vi "run.vi"(8 "error in (no error)":errorcluster, 11 "ScanHeadAK130114ResonanceFlexRIO in":refnum<class "ScanHeadAK130114ResonanceFlexRIO.lvclass">) -> (0 "error out":errorcluster, 3 "ScanHeadAK130114ResonanceFlexRIO out":refnum<class "ScanHeadAK130114ResonanceFlexRIO.lvclass">)   [LabVIEW 2010, in "ScanHeadAK130114ResonanceFlexRIO.lvclass"]
uses:
  ScanHeadAK130114ResonanceFlexRIO.lvclass
  GenericScanHead/GenericScanHead/GenericScanHead.lvclass
  common/classes/ErrorController/ErrorController/ErrorController.lvclass
  Trajectory/GenericTrajectory/GenericTrajectory/GenericTrajectory.lvclass
  internal_trigger_enum.ctl
  main/labview_source/controls/undock_button.ctl
panel:
  in  "button:undock":T1
  in  "Tab Control":enum32{"user", "debug", "about"}(tab)
  in  "number of pulses":u16(ring) items=["0", "1", "2"]
  in  "duration of pulse 2":dbl[unit]
  in  "offset to pulse 2":dbl[unit]
  in  "duration of pulse 1":dbl[unit]
  in  "offset to pulse 1":dbl[unit]
  in  "offset fly back":dbl(slide)=55.301 min=0.001 max=100.0 step=0.1 scale=0.0..100.0
  in  "offset fly forward":dbl(slide)=26.401 min=0.001 max=100.0 step=0.1 scale=0.0..100.0
  in  "scan segment":dbl(slide)=50.001000000000005 min=0.001 max=100.0 step=0.1 scale=0.0..100.0
  in  "modifyButton":bool
  in  "zoom":dbl(slide)=1.5 min=1.0 max=20.0 step=0.1 scale=1.0..20.0
  in  "laser intensity":dbl(slide)=14.5 caption="intensity" min=0.001 max=100.0 step=0.1 scale=0.0..100.0
  in  "stop":bool
  out "event loop error":errorcluster
  out "state machine counter":i32
  out "last trigger":T2
  # "translation"
  # "fov and laser power"
  # "resonance cycle fractions"
  # "ScanHeadAK130114ResonanceFlexRIO"
  # "Author: Andreas Keller, ETH Zurich, Switzerland"
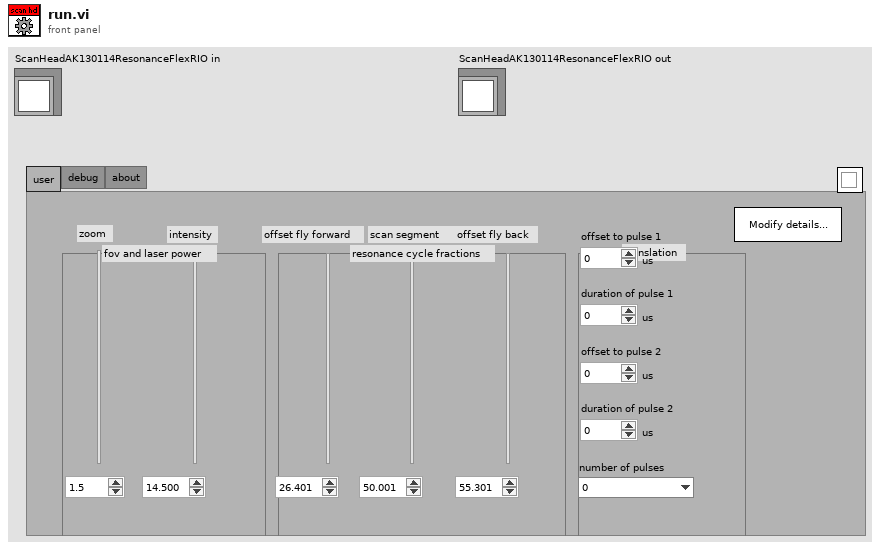
[diagram p1: front panel]
types:
  T1 = typedef "undock_button.ctl" = bool
  T2 = typedef "ScanHeadAK130114ResonanceFlexRIO.lvclass/internal_trigger_enum.ctl" = enum16{"NULL", "initialise", "terminate", "start scanning", "stop scanning", "update", "fetch trajectory"}
  T3 = typedef "top-level_component_type_enum.ctl" = enum16{"undefined", "ImagingMode", "ScanHead", "DAQ", "ImageAssembler", "Display", "DataCollection", "Analyser", "Stimulator", "ExperimentController", "Instrument", "Stage"}
  T4 = typedef "main_trigger_enum.ctl" = enum16{"NULL", "initialise", "terminate", "start", "stop", "change objective", "change experimentController", "change imagingMode", "save notebook", "started saving", "finished saving", "expCtr ready", "expCtr missing", "imgMd ready", "imgMd missing", "scanHd ready", "scanHd missing", "DAQ ready", "DAQ missing", "imgAsm ready", "imgAsm missing", "dataColl ready", "dataColl missing", "display ready", "display missing", "analysr ready", "analysr missing", "instrmnt ready", "instrmnt missing", "stimltr ready", "stimltr missing", "stage ready", "stage missing"}
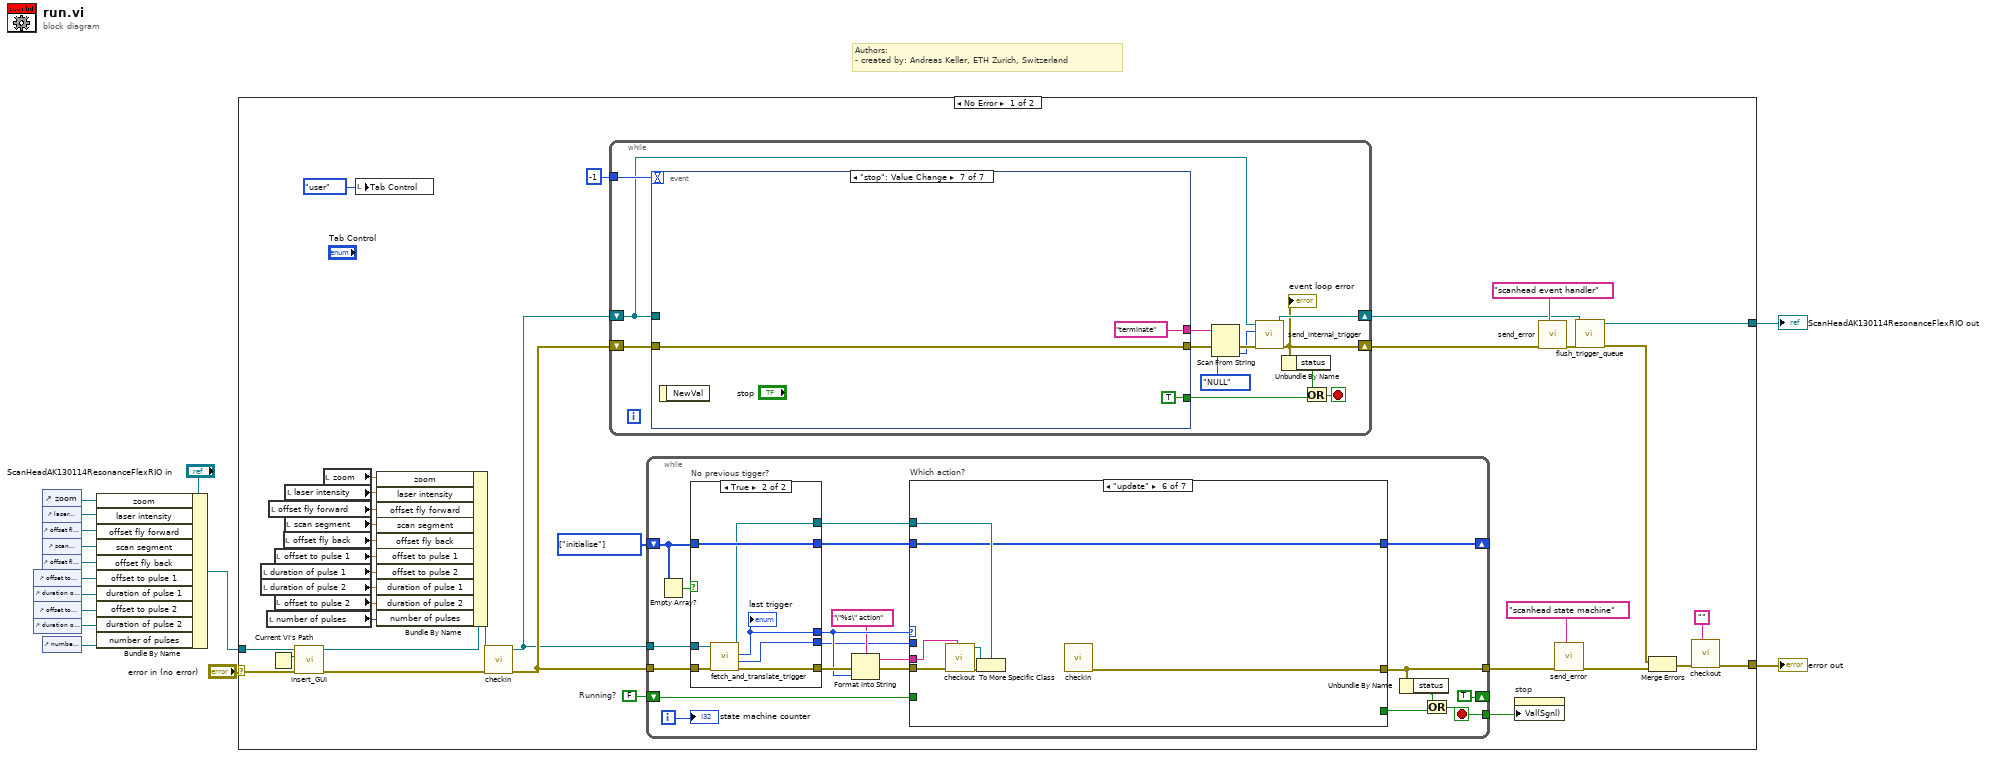
[diagram p0: block diagram]
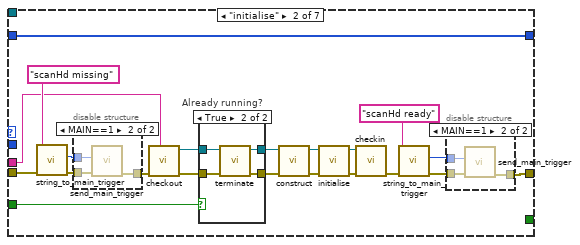
[diagram p3: hidden frame]
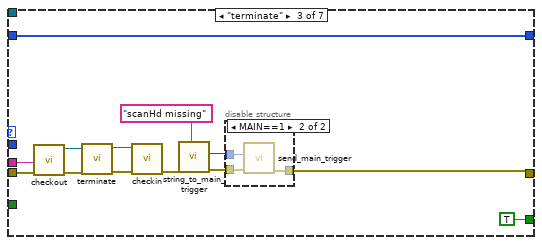
[diagram p7: hidden frame]
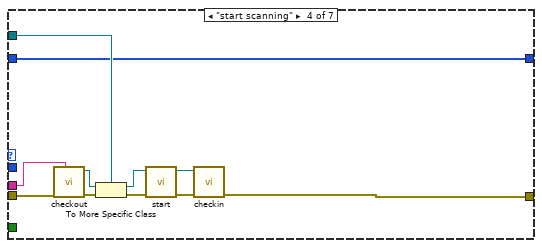
[diagram p9: hidden frame]
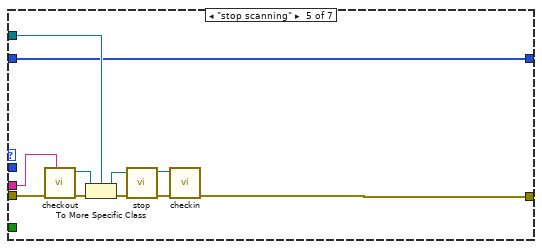
[diagram p10: hidden frame]
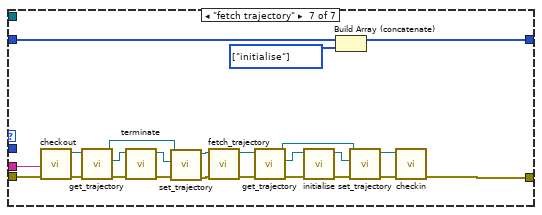
[diagram p11: hidden frame]
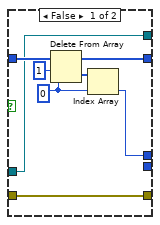
[diagram p12: hidden frame]
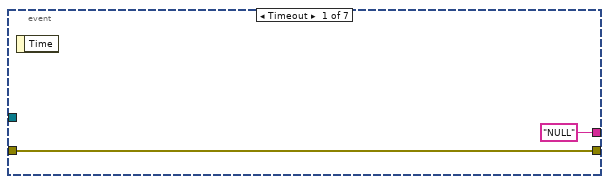
[diagram p13: hidden frame]
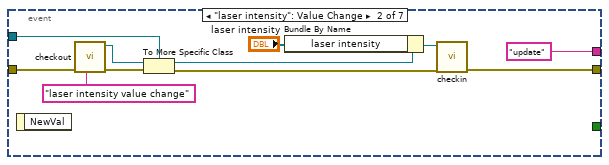
[diagram p14: hidden frame]
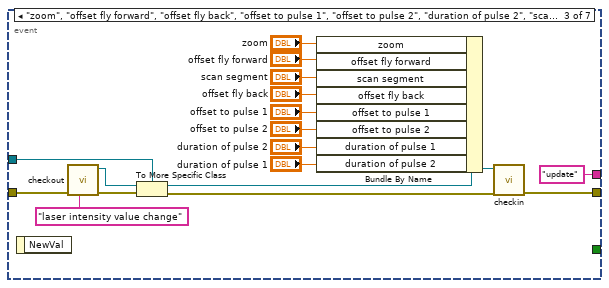
[diagram p15: hidden frame]
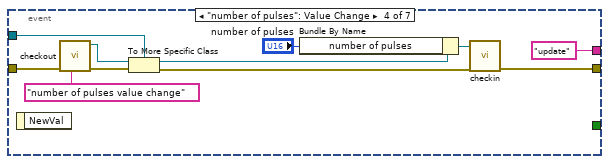
[diagram p16: hidden frame]
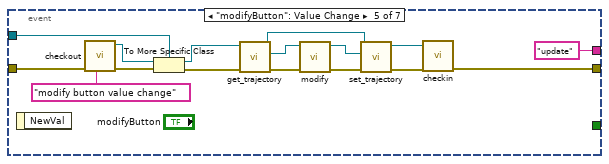
[diagram p17: hidden frame]
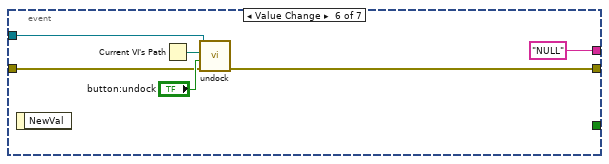
[diagram p18: hidden frame]
diagram:
  # "Authors: \n- created by: Andreas Keller, ETH Zurich, Switzerland"
  n1 = control-ref of="offset to pulse 1"() -> (w6:refnum<vi>)
  n2 = control-ref of="duration of pulse 1"() -> (w5:refnum<vi>)
  n3 = control-ref of="offset to pulse 2"() -> (w4:refnum<vi>)
  n4 = control-ref of="duration of pulse 2"() -> (w3:refnum<vi>)
  n5 = control-ref of="zoom"() -> (w11:refnum<vi>)
  n6 = control-ref of="laser intensity"() -> (w10:refnum<vi>)
  n7 = control-ref of="offset fly forward"() -> (w9:refnum<vi>)
  n8 = control-ref of="scan segment"() -> (w8:refnum<vi>)
  n9 = control-ref of="offset fly back"() -> (w7:refnum<vi>)
  n10 = control-ref of="number of pulses"() -> (w2:refnum<vi>)
  n11 = Bundle By Name(cluster="ScanHeadAK130114ResonanceFlexRIO in", "zoom"=w11, "laser intensity"=w10, "offset fly forward"=w9, "scan segment"=w8, "offset fly back"=w7, "offset to pulse 1"=w6, "duration of pulse 1"=w5, "offset to pulse 2"=w4, "duration of pulse 2"=w3, "number of pulses"=w2) -> (w1:refnum<class "ScanHeadAK130114ResonanceFlexRIO.lvclass">)
  n12 = case shown="No Error" "error in (no error)" {
    selector: "error in (no error)" -> [w48 w273]
    tunnel: w1 -> [w49 w274]
    tunnel: [w27 w274] -> w14
    tunnel: [w24 w273] -> w13
    frame No Error {
      w16 = T2[] [enum."initialise"] items=["NULL", "initialise", "terminate", "start scanning", "stop scanning", "update", "fetch trajectory"]
      w19 = FALSE  # Running?
      n13 = local read "duration of pulse 1"() -> (w40:dbl[unit])
      n14 = local read "duration of pulse 2"() -> (w39:dbl[unit])
      n15 = local read "number of pulses"() -> (w37:u16)
      n16 = local read "offset fly forward"() -> (w44:dbl)
      n17 = Current VI's Path() -> (path=w50:path)
      n18 = local read "offset to pulse 1"() -> (w41:dbl[unit])
      n19 = local read "offset to pulse 2"() -> (w38:dbl[unit])
      n20 = local read "offset fly back"() -> (w42:dbl)
      n21 = local read "scan segment"() -> (w43:dbl)
      n22 = local read "laser intensity"() -> (w45:dbl)
      n23 = call-dynamic "insert_GUI.vi"("error in (no error)"=w48, "VI path"=w50, "GenericComponent in"=w49) -> ("error out"=w36:errorcluster, "GenericComponent out"=w47:refnum<class "ScanHeadAK130114ResonanceFlexRIO.lvclass">)  [unwired: 7 in]
      n24 = local read "zoom"() -> (w46:dbl)
      n25 = local write "Tab Control"(enum32{"user", "debug", "about"}."user" ("Tab Control")) -> ()
      n26 = Bundle By Name(cluster=w47, "zoom"=w46, "laser intensity"=w45, "offset fly forward"=w44, "scan segment"=w43, "offset fly back"=w42, "offset to pulse 1"=w41, "offset to pulse 2"=w40, "duration of pulse 1"=w39, "duration of pulse 2"=w38, "number of pulses"=w37) -> (w35:refnum<class "ScanHeadAK130114ResonanceFlexRIO.lvclass">)
      n27 = call-dynamic "checkin.vi"("error in (no error)"=w36, "GenericScanHead in"=w35) -> ("error out"=w33:errorcluster, "GenericScanHead out"=w32:refnum<class "ScanHeadAK130114ResonanceFlexRIO.lvclass">)  [unwired: 8 in]
      n28 = while {
        tunnel: -1 -> [w205]
        shift-right: [w196] -> w31
        shift-left: w33 -> [w204]
        shift-right: [w198] -> w28
        shift-left: w32 -> [w197]
        stop <- w199 stop-if-true
        n29 = event shown="[6] \"stop\": Value Change" {
          selector: _ -> [_ _ _ _ _ _ _]
          dyn-events: _ -> [_ _ _ _ _ _ _]
          timeout: w205 -> [_ _ _ _ _ _ _]
          tunnel: w204 -> [w206 w211 w232 w238 w261 w267 w272]
          tunnel: [w206 w210 w231 w240 w260 w266 w272] -> w202
          tunnel: ["NULL" "update" "update" "update" "update" "NULL" "terminate"] -> w203
          tunnel: w197 -> [_ w212 w233 w245 w259 w269 _]
          tunnel: [_ _ _ _ _ _ TRUE] -> w194
          event Timeout {
            n30 = event-data() -> ()  [unwired: 1 in, 1 out]
          }
          event "laser intensity": Value Change {
            n31 = event-data() -> ()  [unwired: 1 in, 1 out]
            n32 = call "checkout.vi"("locked by?"="laser intensity value change", "error in (no error)"=w211) -> ("error out"=w216:errorcluster, "GenericScanHead out"=w218:refnum<class "GenericScanHead.lvclass">)  [unwired: 8 in]
            n33 = To More Specific Class(target class=w212, reference=w218, error in=w216) -> (specific class reference=w214:refnum<class "ScanHeadAK130114ResonanceFlexRIO.lvclass">, error out=w215:errorcluster)
            n34 = Bundle By Name(cluster=w214, "laser intensity"="laser intensity") -> (w213:refnum<class "ScanHeadAK130114ResonanceFlexRIO.lvclass">)
            n35 = call-dynamic "checkin.vi"("error in (no error)"=w215, "GenericScanHead in"=w213) -> ("error out"=w210:errorcluster)  [unwired: 8 in, 1 out]
          }
          event "zoom", "offset fly forward", "offset fly back", "offset to pulse 1", "offset to pulse 2", "duration of pulse 2", "scan segment", "duration of pulse 1": Value Change {
            n36 = event-data() -> ()  [unwired: 1 in, 1 out]
            n37 = call "checkout.vi"("locked by?"="laser intensity value change", "error in (no error)"=w232) -> ("error out"=w235:errorcluster, "GenericScanHead out"=w236:refnum<class "GenericScanHead.lvclass">)  [unwired: 8 in]
            n38 = To More Specific Class(target class=w233, reference=w236, error in=w235) -> (specific class reference=w229:refnum<class "ScanHeadAK130114ResonanceFlexRIO.lvclass">, error out=w234:errorcluster)
            n39 = Bundle By Name(cluster=w229, "zoom"="zoom", "offset fly forward"="offset fly forward", "scan segment"="scan segment", "offset fly back"="offset fly back", "offset to pulse 1"="offset to pulse 1", "offset to pulse 2"="offset to pulse 2", "duration of pulse 1"="duration of pulse 2", "duration of pulse 2"="duration of pulse 1") -> (w228:refnum<class "ScanHeadAK130114ResonanceFlexRIO.lvclass">)
            n40 = call-dynamic "checkin.vi"("error in (no error)"=w234, "GenericScanHead in"=w228) -> ("error out"=w231:errorcluster)  [unwired: 8 in, 1 out]
          }
          event "number of pulses": Value Change {
            n41 = event-data() -> ()  [unwired: 1 in, 1 out]
            n42 = call "checkout.vi"("locked by?"="number of pulses value change", "error in (no error)"=w238) -> ("error out"=w247:errorcluster, "GenericScanHead out"=w244:refnum<class "GenericScanHead.lvclass">)  [unwired: 8 in]
            n43 = To More Specific Class(target class=w245, reference=w244, error in=w247) -> (specific class reference=w243:refnum<class "ScanHeadAK130114ResonanceFlexRIO.lvclass">, error out=w246:errorcluster)
            n44 = Bundle By Name(cluster=w243, "number of pulses"="number of pulses") -> (w241:refnum<class "ScanHeadAK130114ResonanceFlexRIO.lvclass">)
            n45 = call-dynamic "checkin.vi"("error in (no error)"=w246, "GenericScanHead in"=w241) -> ("error out"=w240:errorcluster)  [unwired: 8 in, 1 out]
          }
          event "modifyButton": Value Change {
            n46 = event-data() -> ()  [unwired: 1 in, 1 out]
            n47 = call "checkout.vi"("locked by?"="modify button value change", "error in (no error)"=w261) -> ("error out"=w263:errorcluster, "GenericScanHead out"=w258:refnum<class "GenericScanHead.lvclass">)  [unwired: 8 in]
            n48 = To More Specific Class(target class=w259, reference=w258, error in=w263) -> (specific class reference=w257:refnum<class "ScanHeadAK130114ResonanceFlexRIO.lvclass">, error out=w254:errorcluster)
            n49 = call-dynamic "get_trajectory.vi"("error in (no error)"=w254, "GenericScanHead.lvclass in"=w257) -> ("error out"=w256:errorcluster, "trajectory"=w250:refnum<class "GenericTrajectory.lvclass">, "GenericScanHead.lvclass out"=w252:refnum<class "ScanHeadAK130114ResonanceFlexRIO.lvclass">)  [unwired: 7 in]
            n50 = call-dynamic "modify.vi"("error in (no error)"=w256, "GenericTrajectory in"=w250) -> ("error out"=w255:errorcluster, "GenericTrajectory out"=w251:refnum<class "GenericTrajectory.lvclass">)  [unwired: 8 in]
            n51 = call-dynamic "set_trajectory.vi"("error in (no error)"=w255, "trajectory"=w251, "GenericScanHead.lvclass in"=w252) -> ("error out"=w253:errorcluster, "GenericScanHead.lvclass out"=w249:refnum<class "ScanHeadAK130114ResonanceFlexRIO.lvclass">)  [unwired: 7 in]
            n52 = call-dynamic "checkin.vi"("error in (no error)"=w253, "GenericScanHead in"=w249) -> ("error out"=w260:errorcluster)  [unwired: 8 in, 1 out]
          }
          event Value Change {
            n53 = event-data() -> ()  [unwired: 1 in, 1 out]
            n54 = Current VI's Path() -> (path=w265:path)
            n55 = call-dynamic "undock.vi"("error in (no error)"=w267, "undock?"="button:undock", "VI path"=w265, "component in"=w269) -> ("error out"=w266:errorcluster)  [unwired: 6 in, 1 out]
          }
          event "stop": Value Change {
            n56 = event-data() -> ()  [unwired: 1 in, 1 out]
          }
        }
        n57 = Scan From String(input string=w203, error in=w202, default 1=internal_trigger_enum."NULL" ("trigger")) -> (error out=w201:errorcluster, output 1=w195:T2)  [unwired: 2 in, 2 out]
        n58 = call-dynamic "send_internal_trigger.vi"("error in (no error)"=w201, "trigger"=w195, "ScanHeadAK130114ResonanceFlexRIO in"=w197) -> ("error out"=w196:errorcluster, "ScanHeadAK130114ResonanceFlexRIO out"=w198:refnum<class "ScanHeadAK130114ResonanceFlexRIO.lvclass">)  [unwired: 7 in]
        "event loop error" <- w196
        n59 = Unbundle By Name(w196) -> ("status"=w200:bool)
        n60 = Or(x=w200, y=w194) -> (x .or. y?=w199:bool)
      }
      n61 = while {
        tunnel: w33 -> [w70]
        tunnel: [w56] -> w20
        tunnel: w32 -> [w69]
        shift-right: [TRUE ("Running?")] -> _
        shift-left: w19 -> [w59]
        tunnel: [w55] -> w17
        shift-right: [w51] -> _
        shift-left: w16 -> [w53]
        i -> [w60]
        stop <- w55 stop-if-true
        n62 = Empty Array?(array=w53) -> (empty?=w52:bool)
        n63 = case "No previous tigger?" shown="True" w52 {
          tunnel: w70 -> [w179 w191]
          tunnel: [w179 w190] -> w68
          tunnel: w69 -> [w178 w192]
          tunnel: w53 -> [w182 w189]
          tunnel: [w181 w189] -> w62
          tunnel: [w180 w187] -> w66
          tunnel: [_ w188] -> w64
          tunnel: [w178 w186] -> w61
          frame False {
            w183 = 0 ("index")
            n64 = Delete From Array(array=w182, length=1, index=w183) -> (deleted portion=w185:T2[], array with subset deleted=w181:T2[])
            n65 = Index Array(array=w185, index=w183) -> (element=w180:T2)
          }
          frame True {
            n66 = call "fetch_and_translate_trigger.vi"("error in (no error)"=w191, "ScanHeadAK130114ResonanceFlexRIO in"=w192) -> ("error out"=w190:errorcluster, "sender TLC type"=w188:T3, "internal trigger"=w187:T2, "ScanHeadAK130114ResonanceFlexRIO out"=w186:refnum<class "ScanHeadAK130114ResonanceFlexRIO.lvclass">)  [unwired: 6 in]
            "last trigger" <- w187
          }
        }
        n67 = Format Into String(format string="\"%s\" action", error in=w68, w66) -> (resulting string=w63:string, error out=w67:errorcluster)  [unwired: 1 in]
        n68 = case "Which action?" shown="\"update\"" w66 {
          tunnel: w67 -> [w72 w93 w118 w135 w138 w153 w159]
          tunnel: w64 -> [_ _ _ _ _ _ _]
          tunnel: w63 -> [_ w88 w119 w134 w139 w150 w157]
          tunnel: w62 -> [w71 w73 w108 w125 w143 w147 w156]
          tunnel: [w71 w73 w108 w125 w143 w147 w155] -> w51
          tunnel: w61 -> [_ _ _ w132 w144 w152 _]
          tunnel: [w72 w79 w115 w126 w140 w148 w158] -> w56
          tunnel: w59 -> [_ w86 _ _ _ _ _]
          tunnel: [_ _ TRUE _ _ _ _] -> w57
          frame "NULL", Default {
          }
          frame "initialise" {
            n69 = call "string_to_main_trigger.vi"("error in (no error)"=w93, "trigger string"="scanHd missing") -> ("error out"=w90:errorcluster, "main trigger"=w91:T4)  [unwired: 8 in]
            n70 = disable-structure shown="MAIN==1" {
              disable-tunnel: w91 -> [_ w107]
              disable-tunnel: w90 -> [w104 w106]
              disable-tunnel: [w104 w105] -> w89
              frame condition #0 (active) {
              }
              frame condition #1 {
                n71 = call "send_main_trigger.vi"("error in (no error)"=w106, "trigger"=w107) -> ("error out"=w105:errorcluster)  [unwired: 9 in]
              }
            }
            n72 = call "checkout.vi"("locked by?"=w88, "error in (no error)"=w89) -> ("error out"=w87:errorcluster, "GenericScanHead out"=w85:refnum<class "GenericScanHead.lvclass">)  [unwired: 8 in]
            n73 = case "Already running?" shown="True" w86 {
              tunnel: w87 -> [w98 w103]
              tunnel: w85 -> [w99 w102]
              tunnel: [w98 w101] -> w84
              tunnel: [w99 w100] -> w78
              frame False {
              }
              frame True {
                n74 = call-dynamic "terminate.vi"("error in (no error)"=w103, "GenericPlugin in"=w102) -> ("error out"=w101:errorcluster, "GenericPlugin out"=w100:refnum<class "GenericScanHead.lvclass">)  [unwired: 8 in]
              }
            }
            n75 = call-dynamic "construct.vi"("error in (no error)"=w84, "GenericPlugin in"=w78) -> ("error out"=w83:errorcluster, "GenericPlugin out"=w75:refnum<class "GenericScanHead.lvclass">)  [unwired: 8 in]
            n76 = call-dynamic "initialise.vi"("error in (no error)"=w83, "GenericPlugin in"=w75) -> ("error out"=w82:errorcluster, "GenericPlugin out"=w74:refnum<class "GenericScanHead.lvclass">)  [unwired: 8 in]
            n77 = call-dynamic "checkin.vi"("error in (no error)"=w82, "GenericScanHead in"=w74) -> ("error out"=w81:errorcluster)  [unwired: 8 in, 1 out]
            n78 = call "string_to_main_trigger.vi"("error in (no error)"=w81, "trigger string"="scanHd ready") -> ("error out"=w80:errorcluster, "main trigger"=w77:T4)  [unwired: 8 in]
            n79 = disable-structure shown="MAIN==1" {
              disable-tunnel: w77 -> [_ w97]
              disable-tunnel: w80 -> [w94 w96]
              disable-tunnel: [w94 w95] -> w79
              frame condition #0 (active) {
              }
              frame condition #1 {
                n80 = call "send_main_trigger.vi"("error in (no error)"=w96, "trigger"=w97) -> ("error out"=w95:errorcluster)  [unwired: 9 in]
              }
            }
          }
          frame "terminate" {
            n81 = call "checkout.vi"("locked by?"=w119, "error in (no error)"=w118) -> ("error out"=w112:errorcluster, "GenericScanHead out"=w111:refnum<class "GenericScanHead.lvclass">)  [unwired: 8 in]
            n82 = call-dynamic "terminate.vi"("error in (no error)"=w112, "GenericPlugin in"=w111) -> ("error out"=w113:errorcluster, "GenericPlugin out"=w110:refnum<class "GenericScanHead.lvclass">)  [unwired: 8 in]
            n83 = call-dynamic "checkin.vi"("error in (no error)"=w113, "GenericScanHead in"=w110) -> ("error out"=w114:errorcluster)  [unwired: 8 in, 1 out]
            n84 = call "string_to_main_trigger.vi"("error in (no error)"=w114, "trigger string"="scanHd missing") -> ("error out"=w116:errorcluster, "main trigger"=w109:T4)  [unwired: 8 in]
            n85 = disable-structure shown="MAIN==1" {
              disable-tunnel: w109 -> [_ w124]
              disable-tunnel: w116 -> [w121 w123]
              disable-tunnel: [w121 w122] -> w115
              frame condition #0 (active) {
              }
              frame condition #1 {
                n86 = call "send_main_trigger.vi"("error in (no error)"=w123, "trigger"=w124) -> ("error out"=w122:errorcluster)  [unwired: 9 in]
              }
            }
          }
          frame "start scanning" {
            n87 = call "checkout.vi"("locked by?"=w134, "error in (no error)"=w135) -> ("error out"=w133:errorcluster, "GenericScanHead out"=w131:refnum<class "GenericScanHead.lvclass">)  [unwired: 8 in]
            n88 = To More Specific Class(target class=w132, reference=w131, error in=w133) -> (specific class reference=w129:refnum<class "ScanHeadAK130114ResonanceFlexRIO.lvclass">, error out=w130:errorcluster)
            n89 = call-dynamic "start.vi"("error in (no error)"=w130, "ScanHeadAK130114ResonanceFlexRIO in"=w129) -> ("error out"=w128:errorcluster, "ScanHeadAK130114ResonanceFlexRIO out"=w127:refnum<class "ScanHeadAK130114ResonanceFlexRIO.lvclass">)  [unwired: 8 in]
            n90 = call-dynamic "checkin.vi"("error in (no error)"=w128, "GenericScanHead in"=w127) -> ("error out"=w126:errorcluster)  [unwired: 8 in, 1 out]
          }
          frame "stop scanning" {
            n91 = call "checkout.vi"("locked by?"=w139, "error in (no error)"=w138) -> ("error out"=w146:errorcluster, "GenericScanHead out"=w145:refnum<class "GenericScanHead.lvclass">)  [unwired: 8 in]
            n92 = To More Specific Class(target class=w144, reference=w145, error in=w146) -> (specific class reference=w137:refnum<class "ScanHeadAK130114ResonanceFlexRIO.lvclass">, error out=w142:errorcluster)
            n93 = call-dynamic "stop.vi"("error in (no error)"=w142, "ScanHeadAK130114ResonanceFlexRIO in"=w137) -> ("error out"=w141:errorcluster, "ScanHeadAK130114ResonanceFlexRIO out"=w136:refnum<class "ScanHeadAK130114ResonanceFlexRIO.lvclass">)  [unwired: 8 in]
            n94 = call-dynamic "checkin.vi"("error in (no error)"=w141, "GenericScanHead in"=w136) -> ("error out"=w140:errorcluster)  [unwired: 8 in, 1 out]
          }
          frame "update" {
            n95 = call "checkout.vi"("locked by?"=w150, "error in (no error)"=w153) -> ("error out"=w149:errorcluster, "GenericScanHead out"=w151:refnum<class "GenericScanHead.lvclass">)  [unwired: 8 in]
            n96 = To More Specific Class(target class=w152, reference=w151, error in=w149) -> ()  [unwired: 2 out]
            n97 = call-dynamic "checkin.vi"() -> ("error out"=w148:errorcluster)  [unwired: 10 in, 1 out]
          }
          frame "fetch trajectory" {
            w154 = T2[] [enum."initialise"] items=["NULL", "initialise", "terminate", "start scanning", "stop scanning", "update", "fetch trajectory"]
            n98 = call "checkout.vi"("locked by?"=w157, "error in (no error)"=w159) -> ("error out"=w160:errorcluster, "GenericScanHead out"=w164:refnum<class "GenericScanHead.lvclass">)  [unwired: 8 in]
            n99 = call-dynamic "get_trajectory.vi"("error in (no error)"=w160, "GenericScanHead.lvclass in"=w164) -> ("error out"=w165:errorcluster, "trajectory"=w168:refnum<class "GenericTrajectory.lvclass">, "GenericScanHead.lvclass out"=w162:refnum<class "GenericScanHead.lvclass">)  [unwired: 7 in]
            n100 = call-dynamic "terminate.vi"("error in (no error)"=w165, "GenericPlugin in"=w168) -> ("error out"=w167:errorcluster, "GenericPlugin out"=w166:refnum<class "GenericTrajectory.lvclass">)  [unwired: 8 in]
            n101 = call-dynamic "set_trajectory.vi"("error in (no error)"=w167, "trajectory"=w166, "GenericScanHead.lvclass in"=w162) -> ("error out"=w161:errorcluster, "GenericScanHead.lvclass out"=w163:refnum<class "GenericScanHead.lvclass">)  [unwired: 7 in]
            n102 = call-dynamic "fetch_trajectory.vi"("error in (no error)"=w161, "GenericScanHead in"=w163) -> ("error out"=w174:errorcluster, "GenericScanHead out"=w173:refnum<class "GenericScanHead.lvclass">)  [unwired: 8 in]
            n103 = call-dynamic "get_trajectory.vi"("error in (no error)"=w174, "GenericScanHead.lvclass in"=w173) -> ("error out"=w175:errorcluster, "trajectory"=w171:refnum<class "GenericTrajectory.lvclass">, "GenericScanHead.lvclass out"=w172:refnum<class "GenericScanHead.lvclass">)  [unwired: 7 in]
            n104 = call-dynamic "initialise.vi"("error in (no error)"=w175, "GenericPlugin in"=w171) -> ("error out"=w176:errorcluster, "GenericPlugin out"=w170:refnum<class "GenericTrajectory.lvclass">)  [unwired: 8 in]
            n105 = Build Array (concatenate)(w156, w154) -> (w155:T2[])
            n106 = call-dynamic "set_trajectory.vi"("error in (no error)"=w176, "trajectory"=w170, "GenericScanHead.lvclass in"=w172) -> ("error out"=w177:errorcluster, "GenericScanHead.lvclass out"=w169:refnum<class "GenericScanHead.lvclass">)  [unwired: 7 in]
            n107 = call-dynamic "checkin.vi"("error in (no error)"=w177, "GenericScanHead in"=w169) -> ("error out"=w158:errorcluster)  [unwired: 8 in, 1 out]
          }
        }
        n108 = Unbundle By Name(w56) -> ("status"=w58:bool)
        n109 = Or(x=w58, y=w57) -> (x .or. y?=w55:bool)
        "state machine counter" <- w60
      }
      n110 = property on="stop" class="Bool (strict)"("Val(Sgnl)"=w17) -> ()  [unwired: 2 in, 2 out]
      n111 = call "send_error.vi"("additional message"="scanhead event handler" ("locked by?"), "error in (no error)"=w31) -> ("error out"=w29:errorcluster)  [unwired: 9 in]
      n112 = call "send_error.vi"("additional message"="scanhead state machine" ("locked by?"), "error in (no error)"=w20) -> ("error out"=w21:errorcluster)  [unwired: 9 in]
      n113 = call-dynamic "flush_trigger_queue.vi"("error in (no error)"=w29, "GenericToplevelComponent in"=w28) -> ("error out"=w26:errorcluster, "GenericToplevelComponent out"=w27:refnum<class "ScanHeadAK130114ResonanceFlexRIO.lvclass">)  [unwired: 8 in]
      n114 = Merge Errors(w26, w21) -> (w25:errorcluster)
      n115 = call "checkout.vi"("locked by?"="", "error in (no error)"=w25) -> ("error out"=w24:errorcluster)  [unwired: 8 in, 1 out]
    }
    frame Error {
    }
  }
  "error out" <- w13
  "ScanHeadAK130114ResonanceFlexRIO out" <- w14
